vi "Command Done Event.vi"(8 "error in (no error)":errorcluster, 10 "Command In":refnum<class "Command.lvclass">, 11 "Command Handler in":refnum<class "Command Handler.lvclass">) -> (0 "error out":errorcluster)   [LabVIEW 2015, in "Command Handler.lvlib" / "Command Handler.lvclass"]
uses:
  Command Handler.lvclass
  Command Parent/Command.lvclass
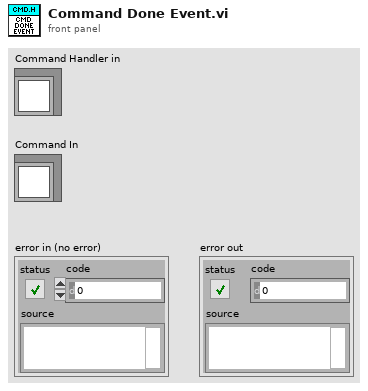
[diagram p1: front panel]
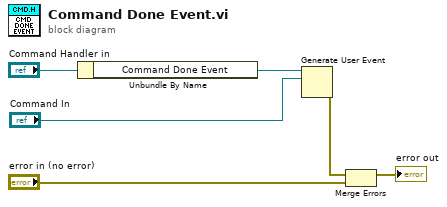
[diagram p0: block diagram]
diagram:
  n1 = Unbundle By Name("Command Handler in") -> ("Command Done Event"=w5:refnum<user-event>)
  n2 = Generate User Event(user event=w5, event data cluster="Command In") -> (error out=w6:errorcluster)  [unwired: 2 in, 1 out]
  n3 = Merge Errors(w6, "error in (no error)") -> (→"error out":errorcluster)
